vi "序列号写入.vi"(8 "Error in":errorcluster caption="Error in (no error)", 10 "序列号":string, 11 "MB session in":refnum<class "MB_Master.lvclass">) -> (0 "error out":errorcluster, 3 "MB session out":refnum<class "MB_Master.lvclass">)   [LabVIEW 2016, in "斯坦道氨氮.lvlib"]
uses:
  <vilib>/Plasmionique/MB Master/MB_Master/MB_Master.lvclass
  <vilib>/Plasmionique/MB Master/MB Master.lvlib
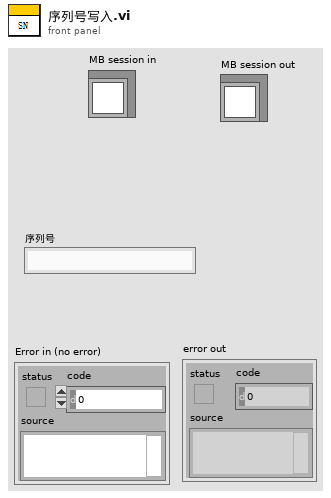
[diagram p1: front panel]
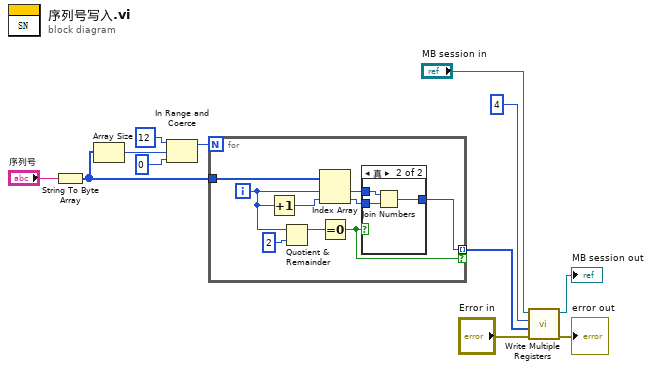
[diagram p0: block diagram]
diagram:
  n1 = String To Byte Array(string="序列号") -> (unsigned byte array=w6:u8[])
  n2 = Array Size(array=w6) -> (size(s)=w4:i32)
  n3 = In Range and Coerce(upper limit=12 ("上限"), x=w4, lower limit=0 ("下限")) -> (coerced(x)=w1:i32)  [unwired: 1 out]
  n4 = for {
    N: w1 -> [_]
    tunnel: w6 -> [w20]
    tunnel: [w21] -> w5 mode=indexing if=w13
    i -> [w17]
    n5 = Increment(x=w17) -> (x+1=w16:i32)
    n6 = Quotient & Remainder(x=w17, y=2) -> (x-y*floor(x/y)=w14:i32)  [unwired: 1 out]
    n7 = Index Array(array=w20, index #1=w17, index #2=w16) -> (element #1=w19:u8, element #2=w15:u8)
    n8 = Equal To 0?(x=w14) -> (x = 0?=w13:bool)
    n9 = case shown="真" w13 {
      tunnel: [_ w24] -> w21
      tunnel: w19 -> [_ w23]
      tunnel: w15 -> [_ w22]
      frame False {
      }
      frame True {
        n10 = Join Numbers(hi=w23, lo=w22) -> ((hi.lo)=w24:u16)
      }
    }
  }
  n11 = call <vilib>:"Write Multiple Registers.vi"("error in (no error)"="Error in", "values"=w5, "starting address"=u16 4, "MB session in"="MB session in") -> ("error out"=→"error out":errorcluster, "MB session out"=→"MB session out":refnum<class "MB_Master.lvclass">)  [unwired: 6 in]
